vi "Add_Columns_to_Results_file.vi"(5 "Edit Raw Data Header Info":bool, 6 "New Value Priority high?":bool, 7 "New Values In":string[](array[string])=[""], 8 "New Chs In":string[](array[string])=[""], 9 "Data filename":path) -> (0 "Filetype":string, 1 "Channel Values Out":string[][](array[string]), 2 "Ch names Out":string[](array[string]), 3 "Data filename out":path, 4 "File Not Changed?":bool)   [LabVIEW 2021]
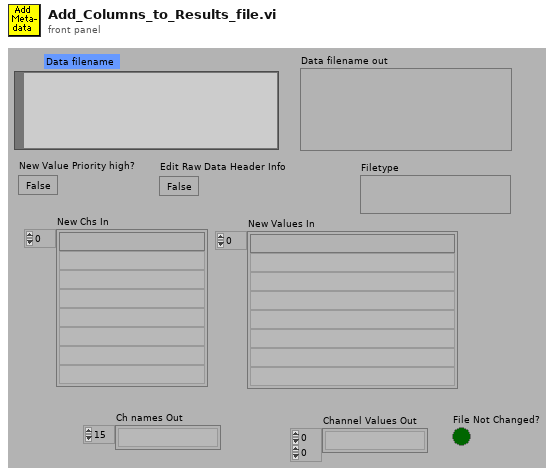
[diagram p1: front panel]
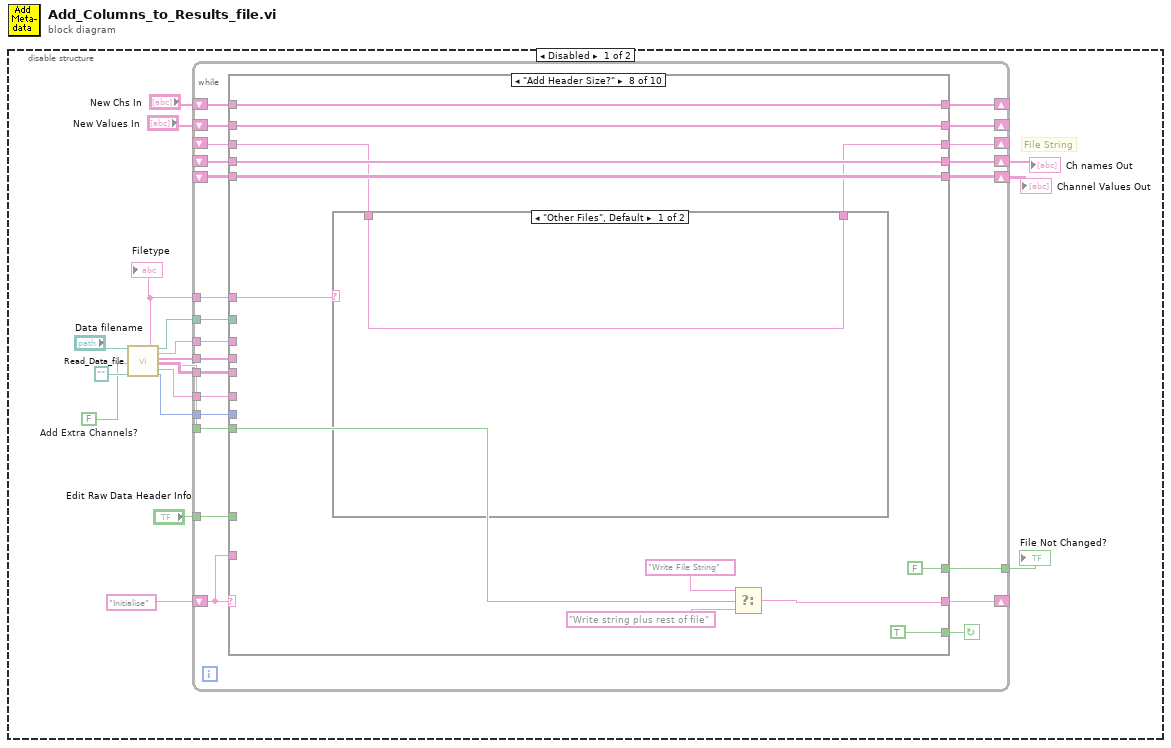
[diagram p0: block diagram]
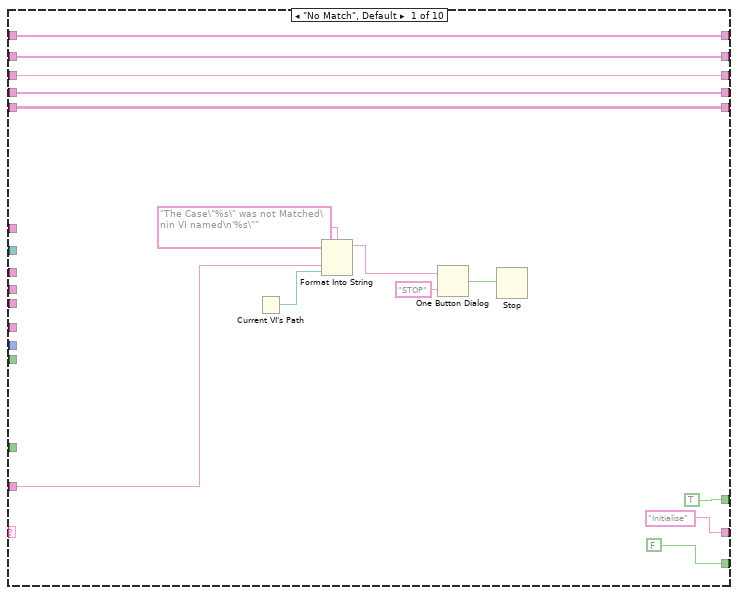
[diagram p2: hidden frame]
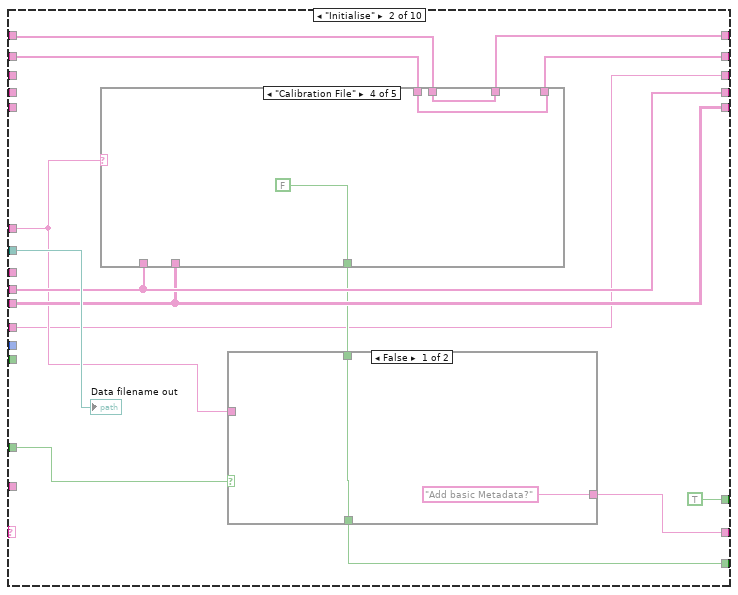
[diagram p3: hidden frame]
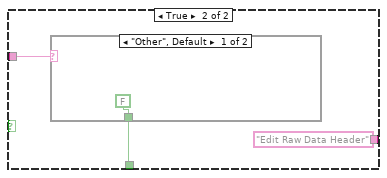
[diagram p4: hidden frame]
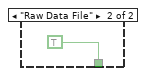
[diagram p5: hidden frame]
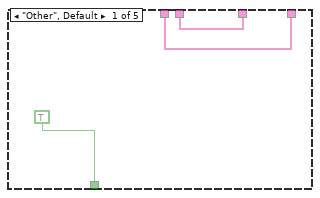
[diagram p6: hidden frame]
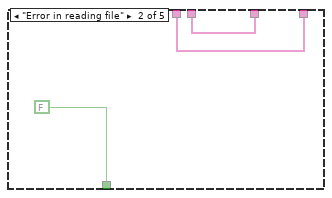
[diagram p7: hidden frame]
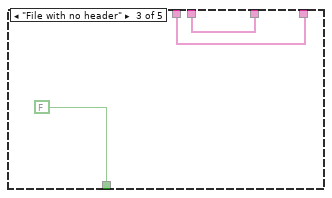
[diagram p8: hidden frame]
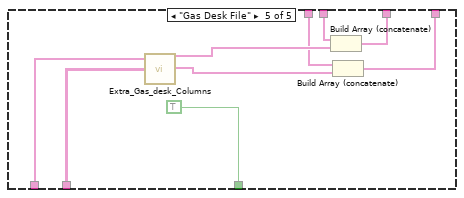
[diagram p9: hidden frame]
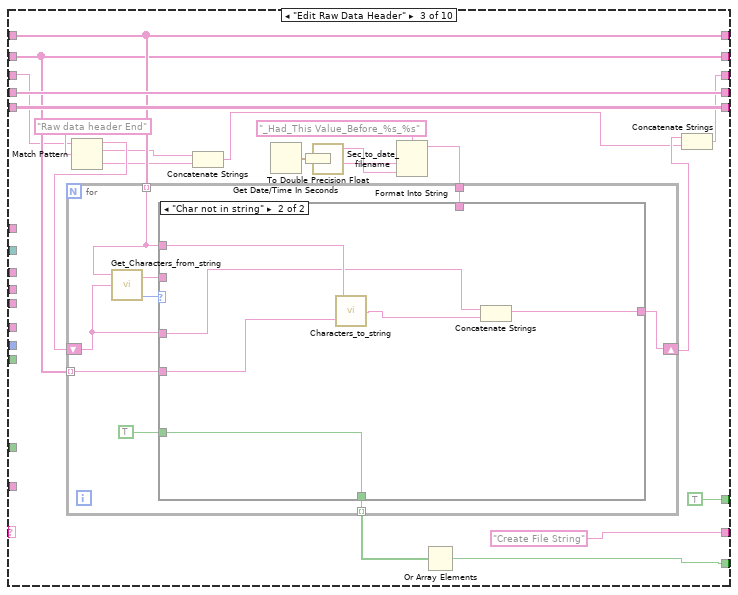
[diagram p10: hidden frame]
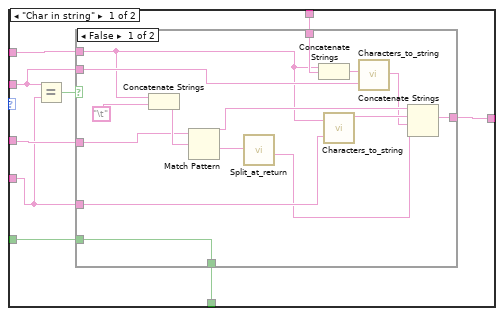
[diagram p11: hidden frame]
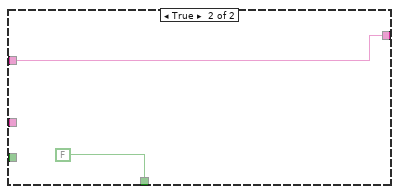
[diagram p12: hidden frame]
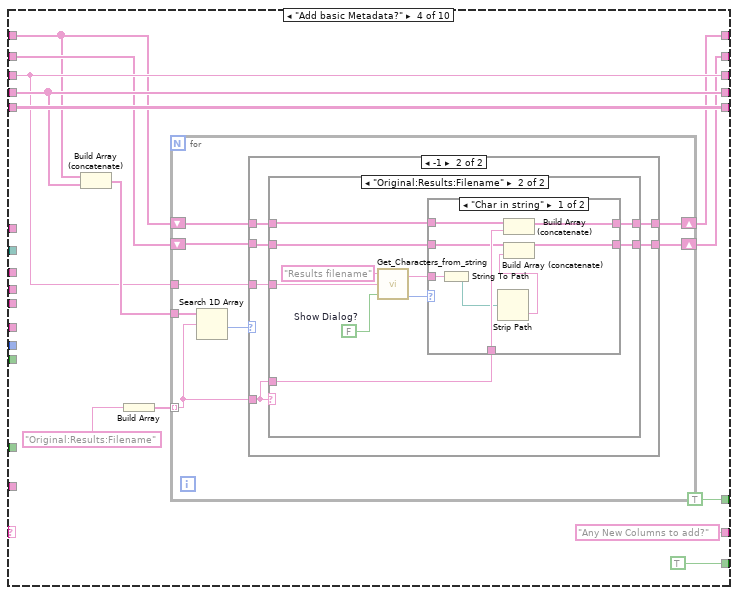
[diagram p13: hidden frame]
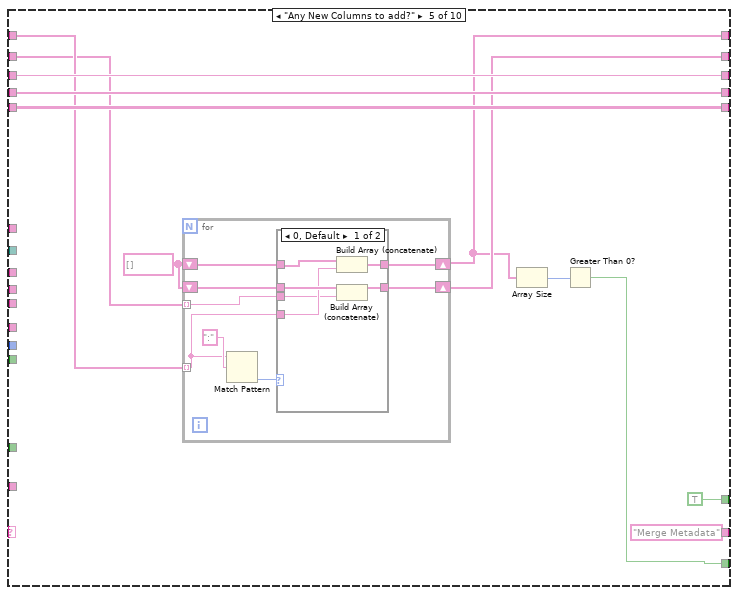
[diagram p17: hidden frame]
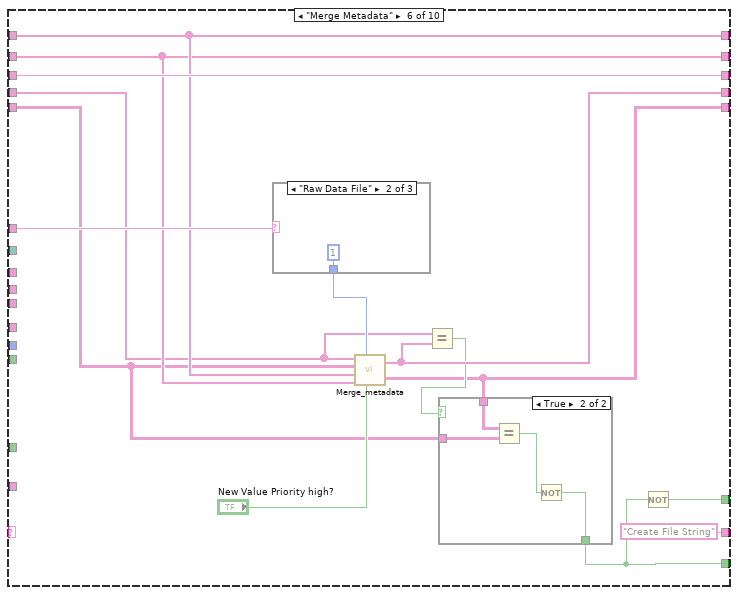
[diagram p19: hidden frame]
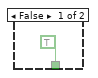
[diagram p20: hidden frame]
diagram:
  n1 = disable-structure shown="Disabled" {
    frame Disabled {
      w16 = FALSE  # Add Extra Channels?
      # "File String"
      n2 = call "Read_Data_file.vi"("Results file"="Data filename", "Add Extra Channels?"=w16, "Template File"=path "") -> ("Filetype"=w11:string, 13:w9, "Results file Out"=w14:path, "String Before"=w10:string, "Ch names Out"=w13:string[], "Channel Values Out"=w12:string[][], "String After"=w8:string, "Start Bytes"=w7:i32)  [unwired: 4 in, 5 out]
      "Filetype" <- w11
      n3 = while {
        tunnel: "Edit Raw Data Header Info" -> [w20]
        shift-left: "New Values In" -> [w22]
        shift-right: [w21] -> _
        shift-left: "New Chs In" -> [w24]
        shift-right: [w23] -> _
        tunnel: w7 -> [w25]
        tunnel: w8 -> [w26]
        tunnel: w9 -> [w27]
        tunnel: w10 -> [w28]
        tunnel: w11 -> [w29]
        tunnel: w12 -> [w30]
        tunnel: w13 -> [w31]
        tunnel: w14 -> [w32]
        shift-left: _ -> [w33]
        shift-right: [w37] -> w5
        shift-left: _ -> [w34]
        shift-right: [w36] -> w6
        shift-left: _ -> [w35]
        shift-right: [w38] -> _
        shift-left: "Initialise" -> [w39]
        shift-right: [w40] -> _
        tunnel: [w19] -> w1
        stop <- w41 continue-if-true
        n4 = case shown="\"Add Header Size?\"" w39 {
          tunnel: [FALSE w56 w99 TRUE w219 w241 TRUE TRUE FALSE FALSE] -> w41
          tunnel: ["Initialise" w61 "Create File String" ("f") "Any New Columns to add?" "Merge Metadata" ("f") "Create File String" ("f") "Add Header Size?" ("f") w283 "End" "End"] -> w40
          tunnel: w39 -> [w50 _ _ _ _ _ _ _ _ _]
          tunnel: [w47 w58 w102 w166 w223 w251 w269 w281 w301 w311] -> w38
          tunnel: [w45 w63 w119 w172 w222 w244 w271 w287 w304 w314] -> w37
          tunnel: [w46 w64 w118 w169 w221 w247 w263 w288 w305 w315] -> w36
          tunnel: w35 -> [w47 _ w108 w166 w223 w251 w265 w282 w301 w311]
          tunnel: w34 -> [w46 _ w118 w169 w221 w246 w263 w288 w305 w315]
          tunnel: w33 -> [w45 _ w119 w172 w222 w243 w271 w287 w304 w314]
          tunnel: w32 -> [_ w69 _ _ _ _ _ _ w302 w312]
          tunnel: w31 -> [_ w64 _ _ _ _ _ _ _ _]
          tunnel: w30 -> [_ w63 _ _ _ _ _ _ _ _]
          tunnel: w29 -> [_ w59 _ _ _ w250 _ w280 _ _]
          tunnel: w28 -> [_ _ _ _ _ _ w270 _ _ _]
          tunnel: w27 -> [_ _ _ _ _ _ _ w284 _ _]
          tunnel: w26 -> [_ w58 _ _ _ _ _ _ _ _]
          tunnel: w25 -> [_ _ _ _ _ _ _ _ _ w310]
          tunnel: w24 -> [w44 w68 w111 w162 w215 w249 w267 w279 w298 w309]
          tunnel: [w44 w67 w111 w165 w213 w249 w267 w279 w298 w309] -> w23
          tunnel: w22 -> [w43 w65 w110 w163 w214 w248 w266 w278 w297 w308]
          tunnel: [w43 w66 w110 w164 w216 w248 w266 w278 w297 w308] -> w21
          tunnel: w20 -> [_ w62 _ _ _ _ _ _ _ _]
          tunnel: [TRUE TRUE TRUE TRUE TRUE w240 FALSE FALSE FALSE FALSE] -> w19
          frame "No Match", Default {
            n5 = Current VI's Path() -> (path=w49:path)
            n6 = Format Into String(format string="The Case\"%s\" was not Matched\nin VI named\n'%s\"" ("Format String"), w50, w49) -> (resulting string=w53:string)  [unwired: 2 in, 1 out]
            n7 = One Button Dialog(message=w53, button name ("OK")="STOP") -> (true=w51:bool)
            n8 = Stop(stop? (T)=w51) -> ()
          }
          frame "Initialise" {
            n9 = case shown="\"Calibration File\"" w59 {
              tunnel: [TRUE FALSE FALSE FALSE TRUE] -> w60
              tunnel: w68 -> [w78 w80 w83 w86 w96]
              tunnel: w65 -> [w77 w81 w84 w87 w94]
              tunnel: [w78 w80 w83 w86 w92] -> w67
              tunnel: [w77 w81 w84 w87 w91] -> w66
              tunnel: w64 -> [_ _ _ _ w90]
              tunnel: w63 -> [_ _ _ _ w89]
              frame "Other", Default {
              }
              frame "Error in reading file" {
              }
              frame "File with no header" {
              }
              frame "Calibration File" {
              }
              frame "Gas Desk File" {
                n10 = call "Extra_Gas_desk_Columns.vi"("Channel Values In"=w89, "Ch names In"=w90) -> ("Extra Values Out"=w93:string[], "Extra Channels Out"=w95:string[])  [unwired: 2 out]
                n11 = Build Array (concatenate)(w96, w95) -> (w92:string[])
                n12 = Build Array (concatenate)(w94, w93) -> (w91:string[])
              }
            }
            n13 = case shown="False" w62 {
              tunnel: ["Add basic Metadata?" "Edit Raw Data Header"] -> w61
              tunnel: [w70 w73] -> w56
              tunnel: w60 -> [w70 _]
              tunnel: w59 -> [_ w74]
              frame False {
              }
              frame True {
                n14 = case shown="\"Other\", Default" w74 {
                  tunnel: [FALSE TRUE] -> w73
                  frame "Other", Default {
                  }
                  frame "Raw Data File" {
                  }
                }
              }
            }
            "Data filename out" <- w69
          }
          frame "Edit Raw Data Header" {
            n15 = Match Pattern(string=w108, regular expression="Raw data header End") -> (before substring=w107:string, match substring=w106:string, after substring=w105:string)  [unwired: 2 out]
            n16 = Concatenate Strings(w106, w105) -> (w103:string)
            n17 = Get Date/Time In Seconds() -> (seconds since 1Jan1904=w98:timestamp)
            n18 = To Double Precision Float(number=w98) -> (double precision float=w113:dbl)
            n19 = call "Sec_to_date_filename.vi"("seconds"=w113) -> ("Year"=w115:string, "Day"=w114:string)  [unwired: 2 out]
            n20 = Format Into String(format string="_Had_This Value_Before_%s_%s" ("Format String"), w114, w115) -> (resulting string=w116:string)  [unwired: 2 in, 1 out]
            n21 = for {
              shift-right: [w123] -> w104
              shift-left: w107 -> [w125]
              tunnel: w111 -> [w126] mode=indexing
              tunnel: w110 -> [w124] mode=indexing
              tunnel: w116 -> [w122]
              tunnel: [w121] -> w100 mode=indexing
              n22 = call "Get_Characters_from_string.vi"("Input string"=w125, "Variable name"=w126) -> ("Status"=w128:enum16{"Char in string", "Char not in string"}, "Value"=w127:string)  [unwired: 1 in]
              n23 = case shown="\"Char not in string\"" w128 {
                tunnel: w126 -> [w135 w160]
                tunnel: w124 -> [w134 w159]
                tunnel: [w136 w158] -> w123
                tunnel: w125 -> [w137 w157]
                tunnel: w127 -> [w132 _]
                tunnel: w122 -> [w131 _]
                tunnel: [w130 w155] -> w121
                tunnel: TRUE -> [w129 w155]
                frame "Char in string" {
                  n24 = Equal?(x=w132, y=w134) -> (x = y?=w133:bool)
                  n25 = case shown="False" w133 {
                    tunnel: w137 -> [w150 w154]
                    tunnel: [w148 w154] -> w136
                    tunnel: w134 -> [w147 _]
                    tunnel: w135 -> [w141 _]
                    tunnel: w132 -> [w143 _]
                    tunnel: w131 -> [w142 _]
                    tunnel: [w138 FALSE] -> w130
                    tunnel: w129 -> [w138 _]
                    frame False {
                      n26 = Concatenate Strings(w141, "\t") -> (w151:string)
                      n27 = Match Pattern(string=w150, regular expression=w151) -> (before substring=w145:string, after substring=w149:string)  [unwired: 3 out]
                      n28 = call "Split_at_return.vi"("String"=w149) -> ("after substring"=w144:string)  [unwired: 1 in, 3 out]
                      n29 = Concatenate Strings(w141, w142) -> (w140:string)
                      n30 = call "Characters_to_string.vi"("Characters to write"=w147, "Label for characters"=w141) -> ("Output string"=w146:string)
                      n31 = call "Characters_to_string.vi"("Characters to write"=w143, "Label for characters"=w140) -> ("Output string"=w139:string)
                      n32 = Concatenate Strings(w145, w146, w139, w144) -> (w148:string)
                    }
                    frame True {
                    }
                  }
                }
                frame "Char not in string" {
                  n33 = call "Characters_to_string.vi"("Characters to write"=w159, "Label for characters"=w160) -> ("Output string"=w156:string)
                  n34 = Concatenate Strings(w157, w156) -> (w158:string)
                }
              }
            }
            n35 = Or Array Elements(Boolean array=w100) -> (logical OR=w99:bool)
            n36 = Concatenate Strings(w104, w103) -> (w102:string)
          }
          frame "Add basic Metadata?" {
            n37 = Build Array (concatenate)(w162, w169) -> (w167:string[])
            n38 = Build Array("Original:Results:Filename") -> (w168:string[])
            n39 = for {
              tunnel: w168 -> [w179] mode=indexing
              tunnel: w167 -> [w180]
              shift-right: [w178] -> w165
              shift-left: w162 -> [w177]
              shift-right: [w175] -> w164
              shift-left: w163 -> [w176]
              tunnel: w166 -> [w174]
              n40 = Search 1D Array(1D array=w180, element=w179) -> (index of element=w181:i32)  [unwired: 1 out]
              n41 = case shown="-1" w181 {
                tunnel: w179 -> [_ w184]
                tunnel: [w183 w189] -> w178
                tunnel: w177 -> [w183 w188]
                tunnel: w176 -> [w182 w187]
                tunnel: [w182 w186] -> w175
                tunnel: w174 -> [_ w185]
                frame 0, Default {
                }
                frame -1 {
                  n42 = case shown="\"Original:Results:Filename\"" w184 {
                    tunnel: [w191 w195] -> w189
                    tunnel: w188 -> [w191 w197]
                    tunnel: w187 -> [w190 w193]
                    tunnel: [w190 w192] -> w186
                    tunnel: w185 -> [_ w200]
                    tunnel: w184 -> [_ w196]
                    frame "Other", Default {
                    }
                    frame "Original:Results:Filename" {
                      w199 = FALSE  # Show Dialog?
                      n43 = call "Get_Characters_from_string.vi"("Show Dialog?"=w199, "Input string"=w200, "Variable name"="Results filename") -> ("Status"=w198:enum16{"Char in string", "Char not in string"}, "Value"=w194:string)
                      n44 = case shown="\"Char in string\"" w198 {
                        tunnel: w197 -> [w209 w211]
                        tunnel: w196 -> [w208 _]
                        tunnel: [w207 w211] -> w195
                        tunnel: w194 -> [w206 _]
                        tunnel: w193 -> [w204 w210]
                        tunnel: [w203 w210] -> w192
                        frame "Char in string" {
                          n45 = String To Path(string=w206) -> (path=w205:path)
                          n46 = Strip Path(path=w205) -> (name=w202:string)  [unwired: 1 out]
                          n47 = Build Array (concatenate)(w209, w208) -> (w207:string[])
                          n48 = Build Array (concatenate)(w204, w202) -> (w203:string[])
                        }
                        frame "Char not in string" {
                        }
                      }
                    }
                  }
                }
              }
            }
          }
          frame "Any New Columns to add?" {
            w217 = string[] []
            n49 = for {
              tunnel: w215 -> [w225] mode=indexing
              shift-right: [w226] -> w213
              shift-left: w217 -> [w229]
              shift-right: [w228] -> w216
              shift-left: w217 -> [w227]
              tunnel: w214 -> [w224] mode=indexing
              n50 = Match Pattern(string=w225, regular expression=":") -> (offset past match=w230:i32)  [unwired: 4 out]
              n51 = case shown="0, Default" w230 {
                tunnel: [w234 w239] -> w226
                tunnel: w229 -> [w237 w239]
                tunnel: [w235 w238] -> w228
                tunnel: w227 -> [w236 w238]
                tunnel: w225 -> [w233 _]
                tunnel: w224 -> [w232 _]
                frame 0, Default {
                  n52 = Build Array (concatenate)(w237, w233) -> (w234:string[])
                  n53 = Build Array (concatenate)(w236, w232) -> (w235:string[])
                }
                frame -1 {
                }
              }
            }
            n54 = Array Size(array=w213) -> (size(s)=w220:i32)
            n55 = Greater Than 0?(x=w220) -> (x > 0?=w219:bool)
          }
          frame "Merge Metadata" {
            n56 = case shown="\"Raw Data File\"" w250 {
              tunnel: [0 ("Comments Row Number") 1 ("Comments Row Number") -1 ("Comments Row Number")] -> w252
              frame "Results File", Default {
              }
              frame "Raw Data File" {
              }
              frame "Gas Desk File" {
              }
            }
            n57 = call "Merge_metadata.vi"("New Value Priority high?"="New Value Priority high?", "Comments Row Number"=w252, "New Values In"=w248, "New Chs In"=w249, "Orig Values In"=w243, "Orig Chs In"=w246) -> ("Channel Values Out"=w244:string[][], "Ch names Out"=w247:string[])
            n58 = Equal?(x=w246, y=w247) -> (x = y?=w245:bool)
            n59 = case shown="True" w245 {
              tunnel: [TRUE w255] -> w241
              tunnel: w244 -> [_ w258]
              tunnel: w243 -> [_ w257]
              frame False {
              }
              frame True {
                n60 = Equal?(x=w258, y=w257) -> (x = y?=w256:bool)
                n61 = Not(x=w256) -> (.not. x?=w255:bool)
              }
            }
            n62 = Not(x=w241) -> (.not. x?=w240:bool)
          }
          frame "Create File String" {
            n63 = call "Ch_names_to_rows.vi"("Channel Names"=w263) -> ("3 Row names"=w262:string[][])
            n64 = Build Array (concatenate)(w262, w271) -> (w272:string[][])
            n65 = Array To Spreadsheet String(array=w272, 3:"%s" ("format string")) -> (spreadsheet string=w274:string)  [unwired: 1 out]
            n66 = call "Remove_end_return.vi"("Input string"=w274) -> ("Output string"=w275:string)
            n67 = Concatenate Strings(w270, w275, w265) -> (w269:string)
          }
          frame "Add Header Size?" {
            n68 = case shown="\"Other Files\", Default" w280 {
              tunnel: w282 -> [w290 w294]
              tunnel: [w290 w291] -> w281
              frame "Other Files", Default {
              }
              frame "Raw Data File" {
                n69 = Match Pattern(string=w294, regular expression="Raw data header End") -> (offset past match=w293:i32)  [unwired: 4 out]
                n70 = call "Raw_Data_File_Start_text.vi"("Header length"=w293) -> ("Start String"=w292:string)
                n71 = Concatenate Strings(w292, w294) -> (w291:string)
              }
            }
            n72 = Select(t="Write File String", s=w284, f="Write string plus rest of file") -> (s? t:f=w283:string)
          }
          frame "Write File String" {
            w300 = FALSE  # append to file? (new file:F)
            w303 = FALSE  # advisory dialog? (display:T)
            n73 = call "Write_Characters_To_File.vi"("file path (dialog if empty)"=w302, "advisory dialog? (display:T)"=w303, "character string"=w301, "append to file? (new file:F)"=w300) -> ()  [unwired: 1 in, 4 out]
          }
          frame "Write string plus rest of file" {
            n74 = stacked-sequence {
              seq-local: [w317 _ _] -> [_ w327 w330]
              tunnel: w312 -> [w318 w328 _]
              tunnel: w311 -> [_ w329 _]
              tunnel: w310 -> [_ w326 _]
              frame #0 {
                n75 = Strip Path(path=w318) -> (stripped path=w325:path, name=w324:string)
                n76 = Concatenate Strings(w324, "_r" ("string")) -> (w323:string)
                n77 = Build Path(base path=w325, name or relative path=w323) -> (appended path=w319:path)
                n78 = call "Copy_with_Check.vi"("Mode"=enum16{"Move", "Copy"}."Move", "Target Path"=w319, "Variable Target?"=FALSE, "Source Path"=w318) -> ("Pathname Out"=w317:path)
              }
              frame #1 {
                n79 = call "Piece_file_Copy.vi"("File Start String"=w329, "Start to copy file at:"=w326, "Source File"=w327, "Target File"=w328) -> ()  [unwired: 1 out]
              }
              frame #2 {
                n80 = Delete(path (use dialog)=w330) -> ()  [unwired: 1 in, 6 out]
              }
            }
          }
        }
      }
      "Ch names Out" <- w6
      "Channel Values Out" <- w5
      "File Not Changed?" <- w1
    }
    frame Enabled {
    }
  }
